vi "FRCts20_Backend_FindUniqueInts.vi"(11 "Input Array":u32[](array[numeric])=[0, 0, 0, 0, 0, 0, 0, 0, 0, 0, 0, 0, 0, 0]) -> (3 "Individual Elements":u32[](array[numeric]))   [LabVIEW 2014]
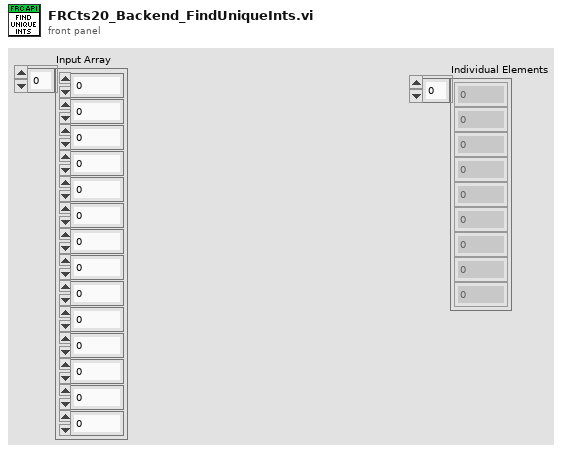
[diagram p1: front panel]
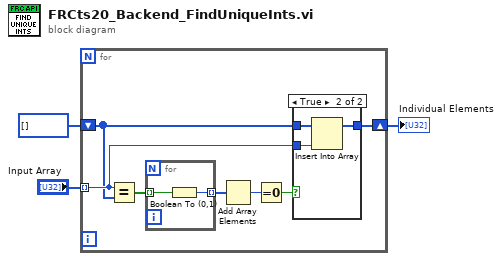
[diagram p0: block diagram]
diagram:
  n1 = for {
    tunnel: "Input Array" -> [w9] mode=indexing
    shift-right: [w10] -> w2
    shift-left: u32[] [] -> [w8]
    n2 = Equal?(x=w9, y=w8) -> (x = y?=w7:bool[])
    n3 = for {
      tunnel: w7 -> [w12] mode=indexing
      tunnel: [w11] -> w6 mode=indexing
      n4 = Boolean To (0,1)(Boolean=w12) -> (0, 1=w11:i16)
    }
    n5 = Add Array Elements(numeric array=w6) -> (sum=w5:i16)
    n6 = Equal To 0?(x=w5) -> (x = 0?=w4:bool)
    n7 = case shown="True" w4 {
      tunnel: w9 -> [_ w16]
      tunnel: [w13 w15] -> w10
      tunnel: w8 -> [w13 w14]
      frame False {
      }
      frame True {
        n8 = Insert Into Array(array=w14, new element=w16) -> (w15:u32[])  [unwired: 1 in]
      }
    }
  }
  "Individual Elements" <- w2
